vi "RescaleAODFrequencyToPixel.vi"(4 "FlipY 2":bool, 6 "FlipX 2":bool, 10 "?":T1={"Calibration Input"=[], "CalibrationResults"={"Center in Pixels"=[374.0120339529387, 375.46592887074246], "Angle"=0.022945275255000355, "Pixels/MHz X"=0.0, "Pixels/MHz Y"=0.0}, "Highlight"=[], "Running Script"=refnum}, 11 "Array 2":dbl[](array[numeric])) -> (3 "Pixels 2":i32[](array[numeric]))   [LabVIEW 2017]
uses:
  TypeDefinitions/ExperimentVariables.ctl
  <vilib>/Analysis/coordinate.llb/2D Cartesian Coordinate Rotation (Scalar).vi
  <vilib>/Analysis/NI_AALPro.lvlib
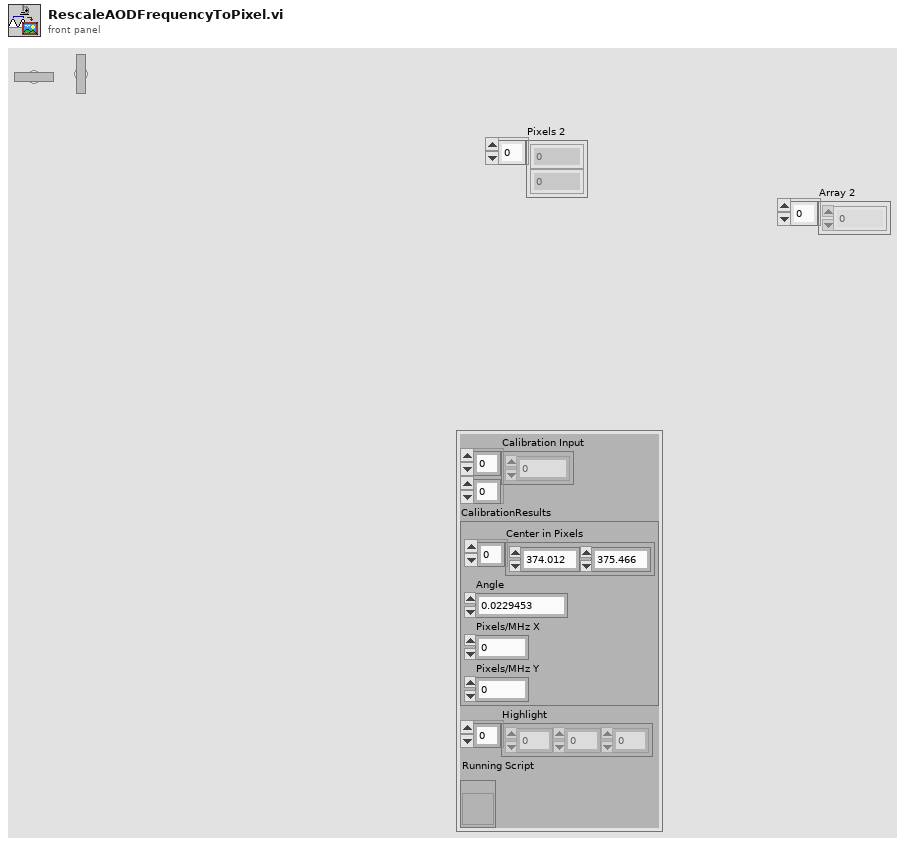
[diagram p1: front panel]
types:
  T1 = typedef "ExperimentVariables.ctl" = cluster{"Calibration Input":i32[][], "CalibrationResults":cluster{"Center in Pixels":dbl[], "Angle":dbl, "Pixels/MHz X":dbl, "Pixels/MHz Y":dbl}, "Highlight":i32[], "Running Script":refnum<vi>}
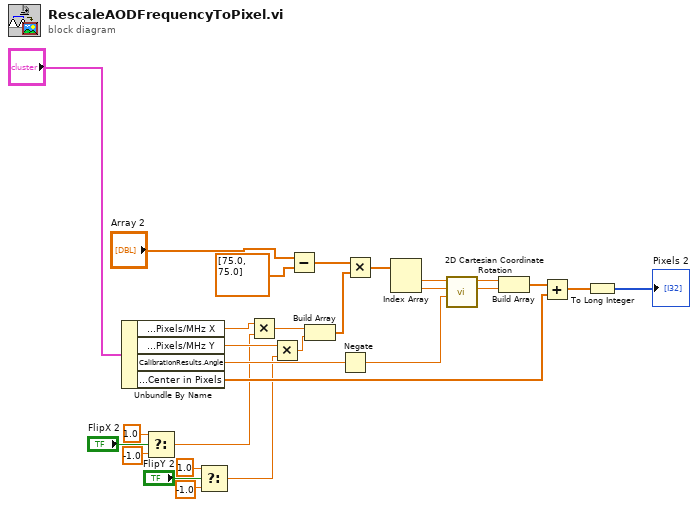
[diagram p0: block diagram]
diagram:
  n1 = Unbundle By Name("?") -> ("CalibrationResults.Pixels/MHz X"=w2:dbl, "CalibrationResults.Pixels/MHz Y"=w4:dbl, "CalibrationResults.Angle"=w16:dbl, "CalibrationResults.Center in Pixels"=w19:dbl[])
  n2 = Select(t=1.0, s="FlipX 2", f=-1.0 ("t")) -> (s? t:f=w1:dbl)
  n3 = Select(t=1.0, s="FlipY 2", f=-1.0 ("t")) -> (s? t:f=w5:dbl)
  n4 = Multiply(x=w2, y=w1) -> (x*y=w3:dbl)
  n5 = Multiply(x=w4, y=w5) -> (x*y=w6:dbl)
  n6 = Subtract(x="Array 2", y=dbl[] [75.0, 75.0]) -> (x-y=w27:dbl[])
  n7 = Build Array(w3, w6) -> (w26:dbl[])
  n8 = Negate(x=w16) -> (-x=w15:dbl)
  n9 = Multiply(x=w27, y=w26) -> (x*y=w25:dbl[])
  n10 = Index Array(array=w25) -> (element #1=w24:dbl, element #2=w23:dbl)  [unwired: 2 in]
  n11 = call-poly <vilib>:"2D Cartesian Coordinate Rotation.vi"("theta"=w15, "y"=w23, "x"=w24) -> ("y out"=w21:dbl, "x out"=w22:dbl)  [unwired: 6 in, 1 out]
  n12 = Build Array(w22, w21) -> (w20:dbl[])
  n13 = Add(x=w20, y=w19) -> (x+y=w18:dbl[])
  n14 = To Long Integer(number=w18) -> (32bit integer=→"Pixels 2":i32[])
